vi "Constructor.vi"(8 "error in (no error)":errorcluster, 11 "Chef in":refnum<class "Chef.lvclass">) -> (0 "error out":errorcluster, 3 "Chef out":refnum<class "Chef.lvclass">)   [LabVIEW 2020, in "Chef.lvclass"]
uses:
  Chef.lvclass
  Oven/Oven.lvclass
  D:/LabVIEW/LabVIEW codes/solutions_and_repetitions/Strategy_pattern/Appliance/Appliance.lvclass
  Chef.lvclass/Chef.ctl
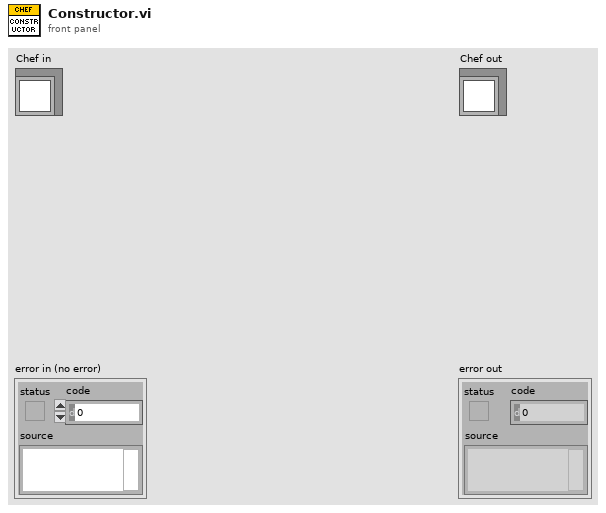
[diagram p1: front panel]
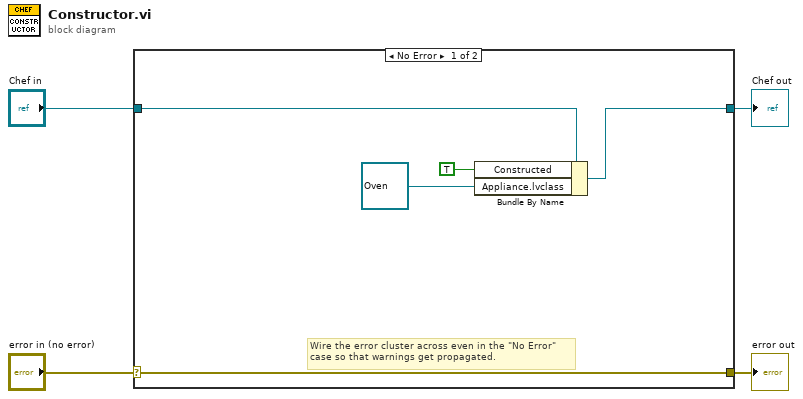
[diagram p0: block diagram]
diagram:
  n1 = case shown="No Error" "error in (no error)" {
    selector: "error in (no error)" -> [w9 w11]
    tunnel: [w9 w11] -> w3
    tunnel: [w7 w10] -> w1
    tunnel: "Chef in" -> [w8 w10]
    frame No Error {
      # "Wire the error cluster across even in the \"No Error\"\ncase so that warnings get propagated."
      n2 = Bundle By Name(cluster=w8, "Constructed"=TRUE, "Appliance.lvclass"=refnum<class "Oven.lvclass"> refnum ("Oven.lvclass")) -> (w7:refnum<class "Chef.lvclass">)
    }
    frame Error {
    }
  }
  "error out" <- w3
  "Chef out" <- w1
